vi "Dialog Box - Progress Message.vi"(0 "Text":string, 3 "error in (no error)":errorcluster, 4 "Show":bool, 5 "Cancel Button (True)":bool=TRUE) -> (8 "Cancel":bool, 10 "error out":errorcluster)   [LabVIEW 2014]
doc: "Displays a dialog box with a cancel button.\n\nThis VI should be called before a long operation with the \"Show\" input set to TRUE, and when the operation completes this VI should be called with \"Show\" set to FALSE."
panel:
  in  "Cancel Button":bool
  out "String":string
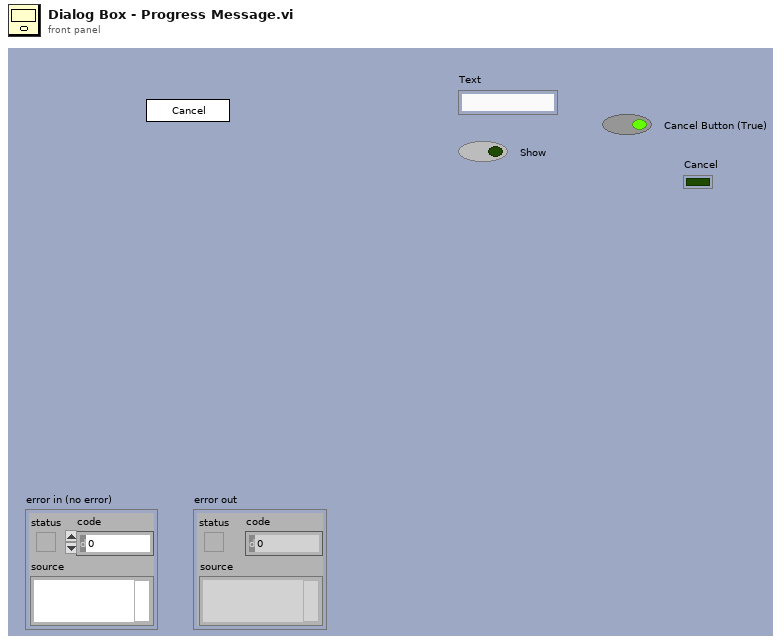
[diagram p1: front panel]
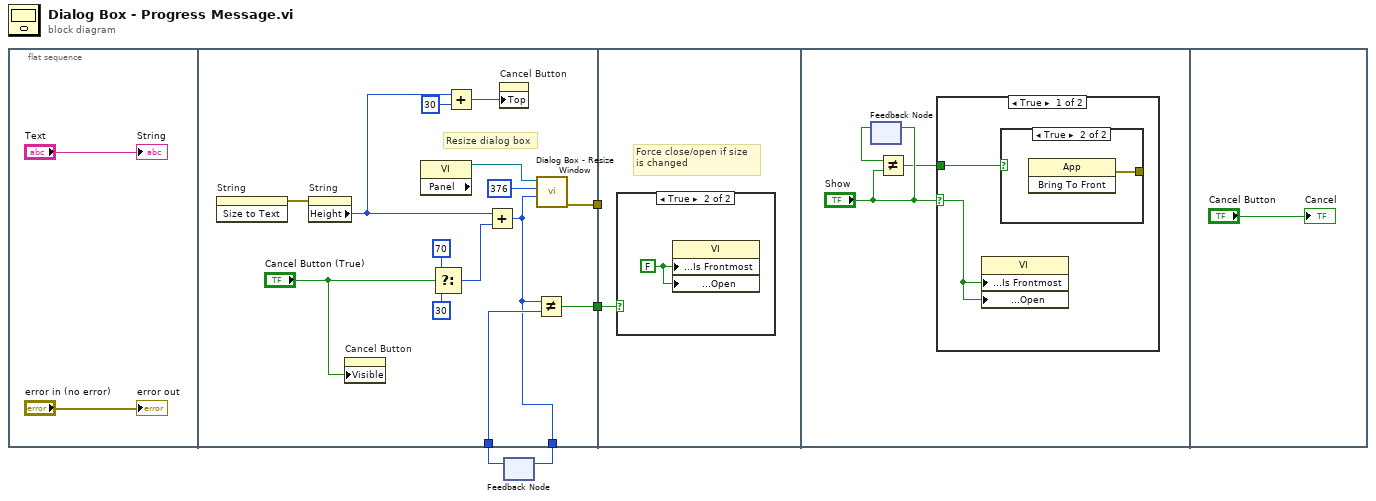
[diagram p0: block diagram]
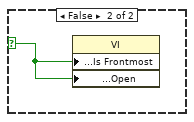
[diagram p4: hidden frame]
diagram:
  n1 = flat-sequence {
    tunnel: [w11] -> w4
    tunnel: [w10] -> w3
    tunnel: [w8] -> w2
    tunnel: w1 -> [w9]
    tunnel: w4 -> [_]
    tunnel: w3 -> [w21]
    frame #0 {
      "String" <- "Text"
      "error out" <- "error in (no error)"
    }
    frame #1 {
      # "Resize dialog box"
      n2 = invoke on="String" class="Str" method="Size to Text"() -> (error out=w20:errorcluster)  [unwired: 3 in, 2 out]
      n3 = property on="String" class="Str"(error in=w20) -> ("Height"=w7:u32)  [unwired: 1 in, 2 out]
      n4 = property on="Cancel Button" class="Bool"("Visible"="Cancel Button (True)") -> ()  [unwired: 2 in, 2 out]
      n5 = property class="VI" props=["Panel"]() -> (reference out=w19:refnum<vi>)  [unwired: 2 in, 2 out]
      n6 = Select(t=u32 70 ("y"), s="Cancel Button (True)", f=u32 30) -> (s? t:f=w14:u32)
      n7 = Add(x=w7, y=u32 30) -> (x+y=w16:u32)
      n8 = Add(x=w7, y=w14) -> (x+y=w8:u32)
      n9 = property on="Cancel Button" class="Bool"("Top"=w16) -> ()  [unwired: 2 in, 2 out]
      n10 = Not Equal?(x=w8, y=w9) -> (x != y?=w10:bool)
      n11 = call "Dialog Box - Resize Window.vi"("Height"=w8, "Width"=i16 376, "reference"=w19) -> ("error out"=w11:errorcluster)  [unwired: 8 in]
    }
    frame #2 {
      # "Force close/open if size\nis changed"
      n12 = case shown="True" w21 {
        frame False {
        }
        frame True {
          w22 = FALSE ("Front Panel Window:Is Frontmost")
          n13 = property class="VI"("Front Panel Window:Is Frontmost"=w22, "Front Panel Window:Open"=w22) -> ()  [unwired: 2 in, 2 out]
        }
      }
    }
    frame #3 {
      n14 = feedback-in #1("Show") -> ()
      n15 = feedback #1() -> (w24:bool)  [unwired: 1 in]
      n16 = Not Equal?(x=w24, y="Show") -> (x != y?=w23:bool)
      n17 = case shown="True" "Show" {
        selector: "Show" -> [w27 w29]
        tunnel: w23 -> [w26 _]
        frame True {
          n18 = property class="VI"("Front Panel Window:Is Frontmost"=w27, "Front Panel Window:Open"=w27) -> ()  [unwired: 2 in, 2 out]
          n19 = case shown="True" w26 {
            tunnel: [_ w28] -> _
            frame False {
            }
            frame True {
              n20 = invoke class="App" method="Bring To Front"() -> (error out=w28:errorcluster)  [unwired: 3 in, 2 out]
            }
          }
        }
        frame False {
          n21 = property class="VI"("Front Panel Window:Is Frontmost"=w29, "Front Panel Window:Open"=w29) -> ()  [unwired: 2 in, 2 out]
        }
      }
    }
    frame #4 {
      "Cancel" <- "Cancel Button"
    }
  }
  n22 = feedback-in #2(w2) -> ()
  n23 = feedback #2() -> (w1:u32)  [unwired: 1 in]
